vi "Command Receiver.vi"() -> ()   [LabVIEW 2023]
uses:
  <vilib>/Platform/TimedLoop/XDataNode/timing_clust.ctl
  <vilib>/Platform/TimedLoop/XDataNode/nitl_modes.ctl
  <vilib>/Platform/TimedLoop/XDataNode/wakeup.ctl
  Type Definitions/Payload Class.ctl
  Type Definitions/Enum - System State.ctl
  Type Definitions/Command TCP State.ctl
  <vilib>/platform/TimedLoop/XDataNode/XDataNode.xnode
  <vilib>/Platform/TimedLoop/XDataNode/XDNodeRunTimeDep.lvlib
panel:
  out "Is Connected":bool
  out "Remote Port":u16
  out "Remote Address":string
  out "Bytes Received":i32
  out "Frames Received":i32
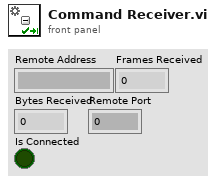
[diagram p1: front panel]
types:
  T1 = typedef "XDNodeRunTimeDep.lvlib/timing_clust.ctl" = cluster{"Expected End [f-1]":u64, "Actual End [f-1]":u64, "Finished Late? [f-1]":bool, "Expected End [i-1]":u64, "Actual End [i-1]":u64, "Finished Late? [i-1]":bool, "Expected Start [i]":u64, "Actual Start [i]":u64, "Expected Start [f]":u64, "Actual Start [f]":u64, "Source Name":string, "Structure Name":string, "Period":i64, "Deadline":i64, "Offset":i64, "Start":i64, "Priority":i32, "Timeout":i32, "Mode":T2, "Wakeup Reason":T3, "Error":errorcluster, "Source Type":string, "Secondary Source Type":string, "Global End Time":u64, "Global Start Time":u64, "Frame Duration":u64, "Iteration Duration":u64, "Assigned CPU":i32, "I/O Scan Engine Mode":u32}
  T2 = typedef "XDNodeRunTimeDep.lvlib/nitl_modes.ctl" = enum32{"No Change", "Process missed periods, maintain original phase", "Discard missed periods, maintain original phase", "Process missed periods, ignore original phase", "Discard missed periods, ignore original phase"}
  T3 = typedef "XDNodeRunTimeDep.lvlib/wakeup.ctl" = enum32{"Normal", "Aborted", "Asynchronous wakeup", "Timing source error", "Timed loop error", "Timeout"}
  T4 = typedef "Data Frame.ctl" = cluster{"Frame Header":T5, "Payload":string, "CRC":u32}
  T5 = typedef "Data Frame Header.ctl" = cluster{"Sync":u32, "Time":dbl, "Nanosecond Counter":i64, "Payload Class":T6, "Payload ID":u16, "Counter":i32, "Options":u32, "Source":T7, "Destination":T7}
  T6 = typedef "Payload Class.ctl" = enum16{"System State", "Parameters", "Metadata", "Software Monitor", "Data", "Commands"}
  T7 = typedef "Device.ctl" = enum32{"None", "Exec", "Aux1", "Aux2", "Aux3"}
  T8 = typedef "Command TCP State.ctl" = cluster{"Is Connected":bool, "Remote Address":string, "Remote Port":u16, "Total Frames Sent":i32, "Total Bytes Sent":i32}
  T9 = typedef "Enum - System State.ctl" = enum16{"System Time", "Telemetry TCP State", "Writeable Drive State", "Command TCP State", "Network Adapter State", "Discovery Engine State", "Disk State"}
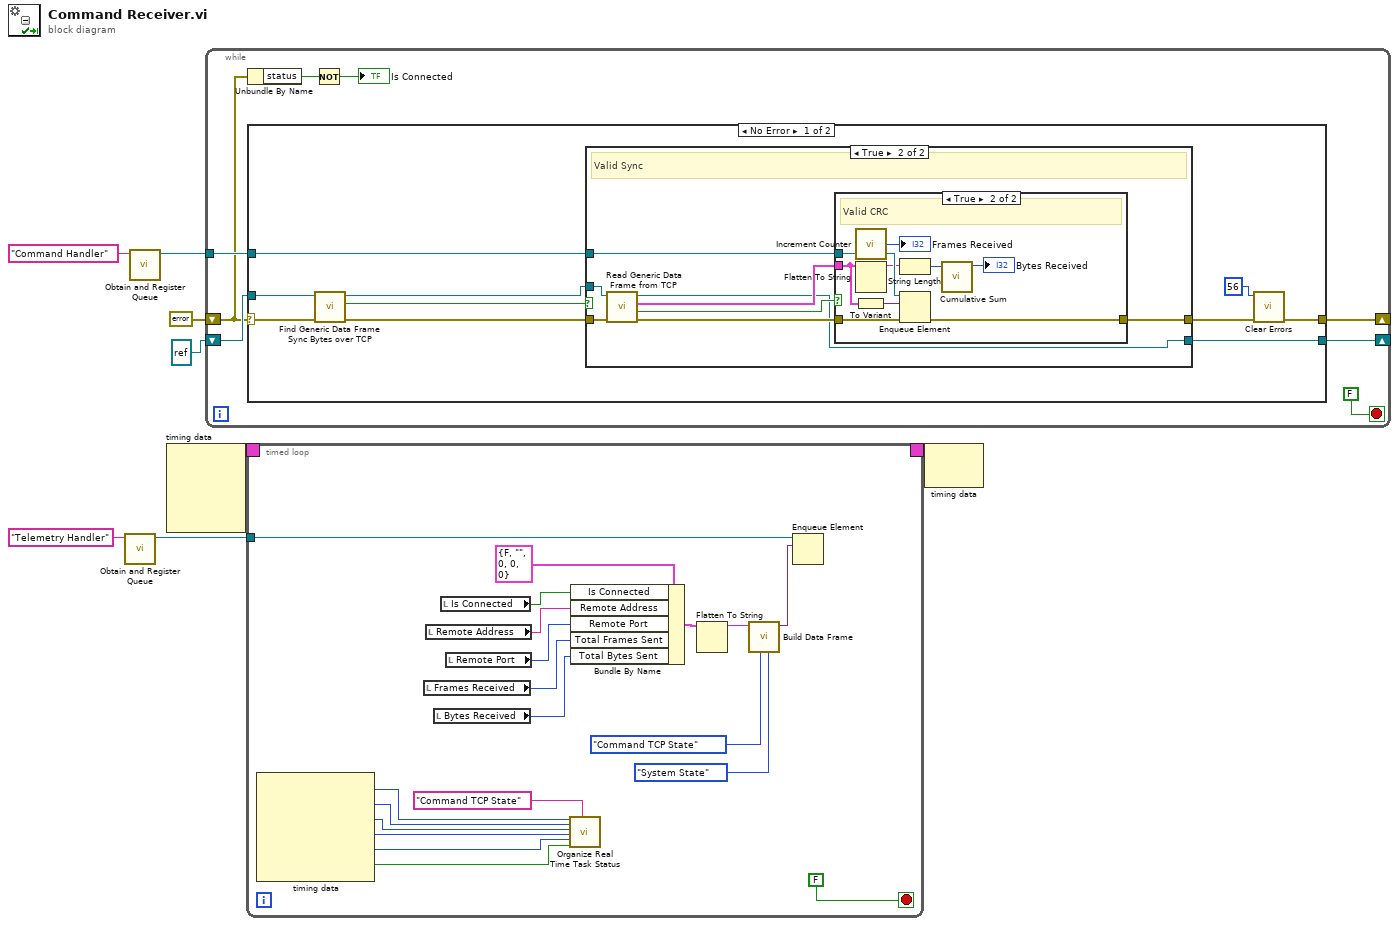
[diagram p0: block diagram]
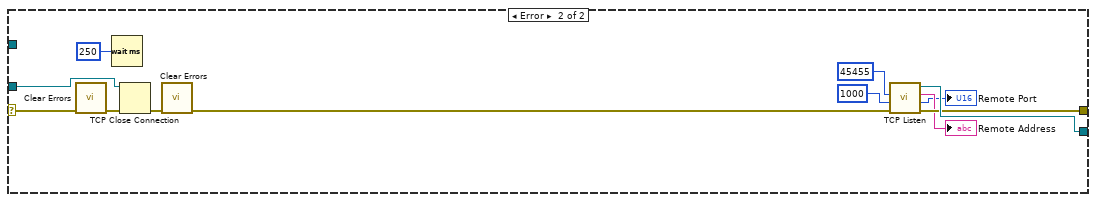
[diagram p4: hidden frame]
diagram:
  n1 = call "Obtain and Register Queue.vi"("Queue Name (unnamed)"="Telemetry Handler" ("name (unnamed)")) -> ("Queue Reference"=w3:refnum<queue>)  [unwired: 9 in, 1 out]
  n2 = call "Obtain and Register Queue.vi"("Queue Name (unnamed)"="Command Handler" ("name (unnamed)")) -> ("Queue Reference"=w6:refnum<queue>)  [unwired: 9 in, 1 out]
  n3 = node-c288() -> (w5:T1)  [unwired: 4 in]
  n4 = while {
    shift-right: [w12] -> _
    shift-left: errorcluster {"status"=TRUE, "code"=0, "source"=""} ("error in (no error)") -> [w11]
    shift-right: [w16] -> _
    shift-left: refnum<k5> refnum ("connection ID") -> [w15]
    tunnel: w6 -> [w13]
    stop <- FALSE stop-if-true
    n5 = Unbundle By Name(w11) -> ("status"=w10:bool)
    n6 = case shown="No Error" w11 {
      selector: w11 -> [w26 w58]
      tunnel: [w17 w50] -> w12
      tunnel: [w23 w51] -> w16
      tunnel: w15 -> [w25 w54]
      tunnel: w13 -> [w20 _]
      frame No Error {
        n7 = call "Find Generic Data Frame Sync Bytes over TCP.vi"("error in (no error)"=w26, "TCP Network Connection in"=w25) -> ("error out"=w22:errorcluster, "Valid Sync"=w21:bool, "TCP Network Connection out"=w24:refnum<k5>)  [unwired: 7 in]
        n8 = case shown="True" w21 {
          tunnel: w24 -> [w28 w36]
          tunnel: [w28 w29] -> w23
          tunnel: w22 -> [w27 w35]
          tunnel: [w27 w30] -> w18
          tunnel: w20 -> [_ w32]
          frame False {
            # "Invalid Sync"
          }
          frame True {
            # "Valid Sync"
            n9 = call "Read Generic Data Frame from TCP.vi"("error in (no error)"=w35, "TCP Network Connection in"=w36) -> ("error out"=w31:errorcluster, "Valid CRC"=w33:bool, "Frame Received"=w34:T4, "TCP Network Connection out"=w29:refnum<k5>)  [unwired: 6 in]
            n10 = case shown="True" w33 {
              tunnel: w34 -> [_ w41]
              tunnel: w32 -> [_ w46]
              tunnel: w31 -> [w37 w45]
              tunnel: [w37 w44] -> w30
              frame False {
                # "Invalid CRC"
              }
              frame True {
                # "Valid CRC"
                n11 = call "Increment Counter.vi"() -> ("Count"=→"Frames Received":i32)  [unwired: 5 in]
                n12 = Flatten To String(anything=w41) -> (data string=w40:string)  [unwired: 3 in, 2 out]
                n13 = To Variant(anything=w41) -> (Variant=w43:variant)
                n14 = String Length(string=w40) -> (length=w39:i32)
                n15 = Enqueue Element(queue=w46, element=w43, error in (no error)=w45) -> (error out=w44:errorcluster)  [unwired: 1 in, 2 out]
                n16 = call "Cumulative Sum.vi"("Value In"=w39) -> ("Cumulative Sum"=→"Bytes Received":i32)  [unwired: 9 in, 1 out]
              }
            }
          }
        }
        n17 = call <vilib>:"Clear Errors.vi"("error in (no error)"=w18, "specific error code to clear (0: all)"=56) -> ("error out"=w17:errorcluster)  [unwired: 4 in, 1 out]
      }
      frame Error {
        n18 = call <vilib>:"Clear Errors.vi"("error in (no error)"=w58) -> ("error out"=w56:errorcluster)  [unwired: 5 in, 1 out]
        n19 = Wait (ms)(milliseconds to wait=u32 250) -> ()  [unwired: 1 out]
        n20 = TCP Close Connection(connection ID=w54, error in (no error)=w56) -> (error out=w55:errorcluster)  [unwired: 1 in, 1 out]
        n21 = call <vilib>:"Clear Errors.vi"("error in (no error)"=w55) -> ("error out"=w47:errorcluster)  [unwired: 5 in, 1 out]
        n22 = call <vilib>:"TCP Listen.vi"("error in (no error)"=w47, "timeout ms (wait forever: -1)"=1000, "port"=u16 45455) -> ("error out"=w50:errorcluster, "remote port"=→"Remote Port":u16, "remote address"=→"Remote Address":string, "connection ID"=w51:refnum<k5>)  [unwired: 4 in, 1 out]
      }
    }
    n23 = Not(x=w10) -> (.not. x?=→"Is Connected":bool)
  }
  n24 = timed-loop {
    timing: w5 -> [_]
    timing-out: [_] -> w4
    tunnel: w3 -> [w67]
    stop <- FALSE stop-if-true
    n25 = node-c288() -> (w76:i32, w75:i32, w74:i64, w73:i64, w72:i64, w71:bool)  [unwired: 1 in]
    n26 = local read "Frames Received"() -> (w62:i32)
    n27 = local read "Remote Address"() -> (w64:string)
    n28 = local read "Bytes Received"() -> (w61:i32)
    n29 = local read "Is Connected"() -> (w60:bool)
    n30 = local read "Remote Port"() -> (w63:u16)
    n31 = call "Organize Real Time Task Status.vi"("Priority"=w76, "Processor"=w75, "Offset"=w74, "Iteration Duration"=w73, "Period"=w72, "Finished Late? [i-1]"=w71, "Task Name"="Command TCP State") -> ()  [unwired: 12 in, 1 out]
    n32 = Bundle By Name(cluster=T8 {"Is Connected"=FALSE, "Remote Address"="", "Remote Port"=0, "Total Frames Sent"=0, "Total Bytes Sent"=0} ("Command TCP State"), "Is Connected"=w60, "Remote Address"=w64, "Remote Port"=w63, "Total Frames Sent"=w62, "Total Bytes Sent"=w61) -> (w66:T8)
    n33 = Flatten To String(anything=w66) -> (data string=w69:string)  [unwired: 3 in, 2 out]
    n34 = call "Build Data Frame.vi"("Payload Class (Data)"=Payload_Class."System State", "Payload ID (0)"=Enum_-_System_State."Command TCP State" ("System State"), "Payload (Empty String)"=w69) -> ("Frame"=w68:variant)  [unwired: 7 in, 1 out]
    n35 = Enqueue Element(queue=w67, element=w68) -> ()  [unwired: 2 in, 3 out]
  }
  n36 = node-c288(w4) -> ()  [unwired: 1 out]
